vi "UUT Emulation Global.vi"() -> ()   [LabVIEW 2013]
panel:
  in  "Emulated Packet Error Rate":dbl=30.8
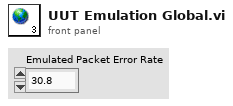
[diagram p1: front panel]
diagram:
